vi "纳清浊度电极校准.vi"() -> ()   [LabVIEW 2016, in "斯坦道多参数.lvlib"]
uses:
  <vilib>/Utility/miscctls.llb/LVPointTypeDef.ctl
  <vilib>/Utility/miscctls.llb/LVPositionTypeDef.ctl
  <vilib>/Analysis/NI_AALBase.lvlib
panel:
  out "滤波设定":sgl
  out "第三点信号值":dbl
  out "第二点信号值":dbl
  out "第一点信号值":dbl
  in  "量程":u16(ring) items=["0-100", "0-500", "0-2000", "0-4000"]
  out "报警信息":string
  out "通讯状态":string
  out "第三点校准值":dbl
  out "标液3":sgl
  out "第二点校准值":dbl
  out "第一点校准值":dbl
  in  "校准停止":bool
  in  "校准启动":bool
  in  "校准模式":u16(ring)=1 items=["两点校准", "单点校准", "三点校准"]
  out "最小值":sgl format="%#.2f"
  out "最大值":sgl format="%#.2f"
  out "波形图表":dbl(graph) caption="历史曲线"
  out "mean":dbl caption="均值" format="%#.2f"
  out "standard deviation":dbl caption="标准差" format="%#.2f"
  out "变异系数":dbl format="%#.6f"
  out "测量值":sgl format="%#.2f"
  out "提示":string
  out "标液2":sgl
  out "标液1":sgl
  out "原始光强数值":u16 caption="信号值"
  out "温度":dbl format="%#.2f"
  # "浊度电极设定"
  # "℃"
  # "NTU"
  # "NTU"
  # "请选择校准模式:"
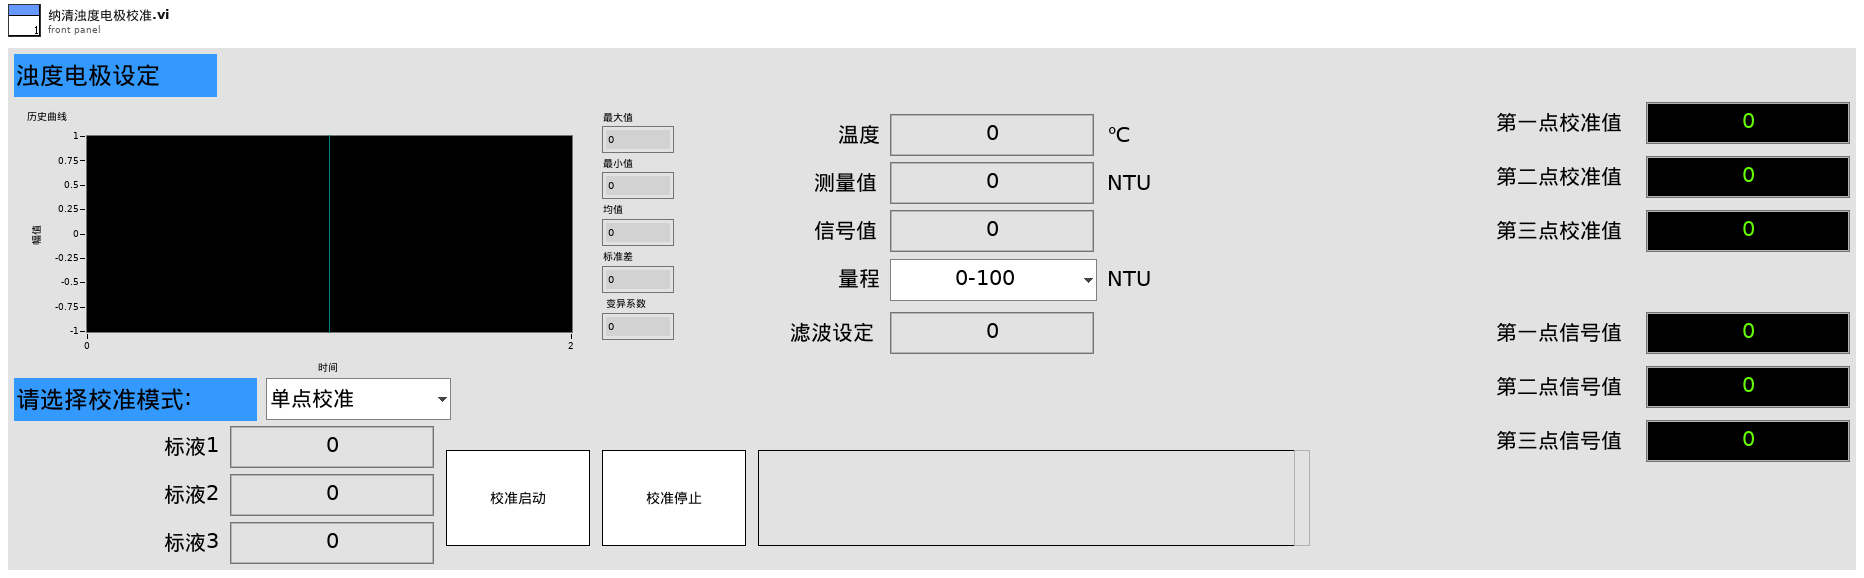
[diagram p1: front panel]
types:
  T1 = enum16{"pH", "DO", "Cond", "Turb", "ORP", "叶绿素a", "藻密度"}
  T2 = typedef "LVPointTypeDef.ctl" = cluster{"Horizontal":i16, "Vertical":i16}
  T3 = cluster{"报警码":u16, "浊度数值 NTU":sgl, "温度数据":sgl, "原始光强数值":u16, "量程":u16, "平均次数":u16, "清扫模式":u16, "清扫次数":u16, "清扫间隔分钟":u16, "0X000B_NC":string, "产品名称":string, "序列号":string, "硬件版本":string, "软件版本":string, "通讯地址":u16, "波特率":u16, "设备类型":u16, "0X0026_NC":string, "校准量程":u16, "第一点原始光强":u16, "第一点校准数据":sgl, "第二点原始光强":u16, "第二点校准数据":sgl, "第三点原始光强":u16, "第三点校准数据":sgl, "探头校准命令":u16, "温度校准参数":sgl, "温度校准命令":u16}
  T4 = cluster{"pH":u32, "DO":u32, "Cond":u32, "Turb":u32, "叶绿素a":u32, "藻密度":u32, "ORP":u32}
  T5 = typedef "LVPositionTypeDef.ctl" = cluster{"Left":i32, "Top":i32}
  T6 = enum8{"Enabled", "Disabled", "Disabled and Grayed Out"}
  T7 = cluster{"报警码":u16, "叶绿素a":sgl, "温度数据":sgl, "原始光强数值":u16, "量程":u16, "平均次数":u16, "清扫模式":u16, "清扫次数":u16, "清扫间隔分钟":u16, "0X000B_NC":string, "产品名称":string, "序列号":string, "硬件版本":string, "软件版本":string, "通讯地址":u16, "波特率":u16, "设备类型":u16, "0X0026_NC":string, "校准量程":u16, "第一点原始光强":u16, "第一点校准数据":sgl, "第二点原始光强":u16, "第二点校准数据":sgl, "第三点原始光强":u16, "第三点校准数据":sgl, "探头校准命令":u16, "温度校准参数":sgl, "温度校准命令":u16}
  T8 = cluster{"ph":bool, "DO":bool, "Cond":bool, "Turb":bool, "叶绿素a":bool, "藻密度":bool, "ORP":bool}
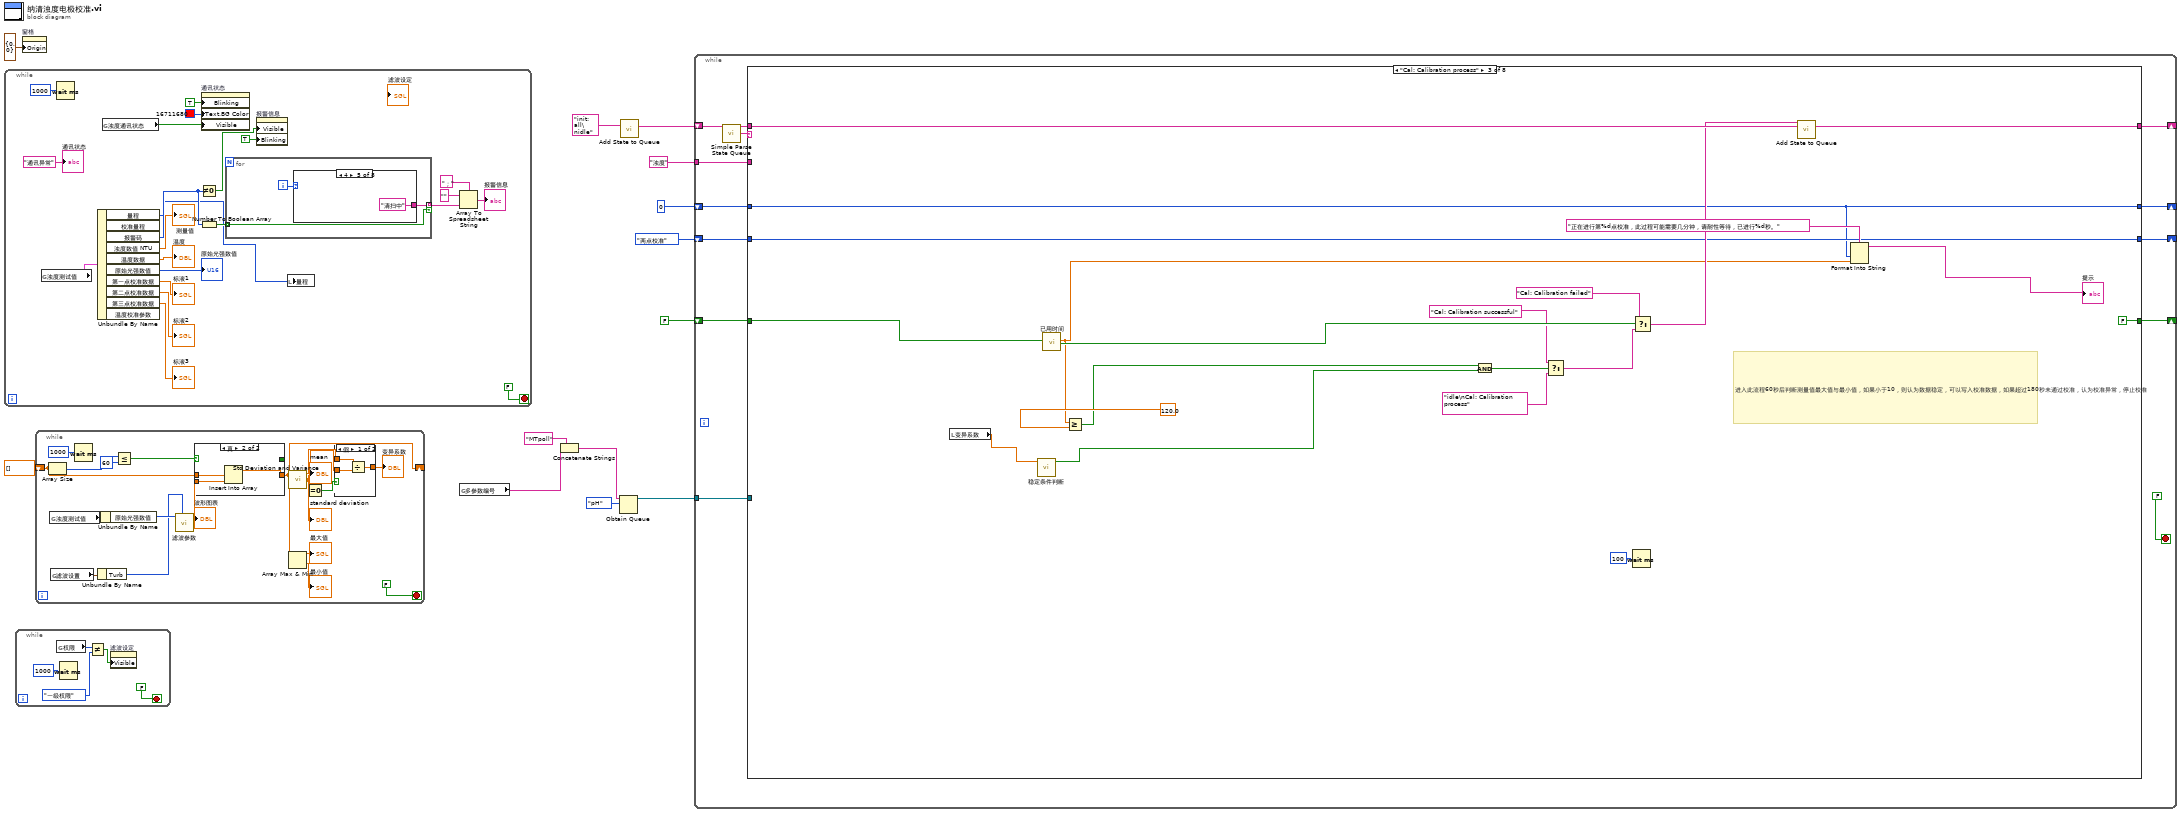
[diagram p0: block diagram]
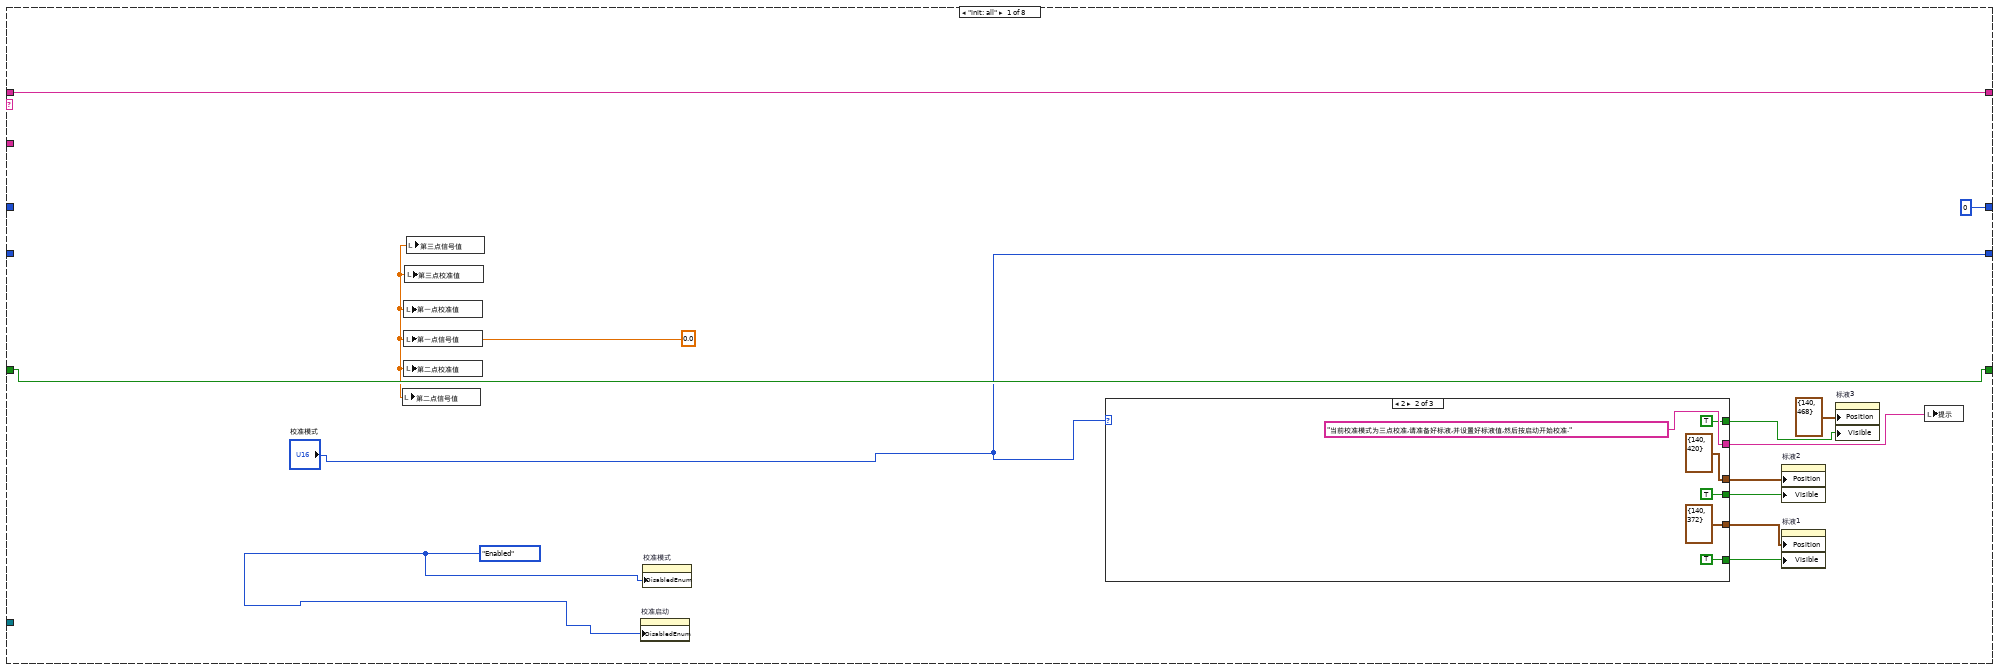
[diagram p2: hidden frame]
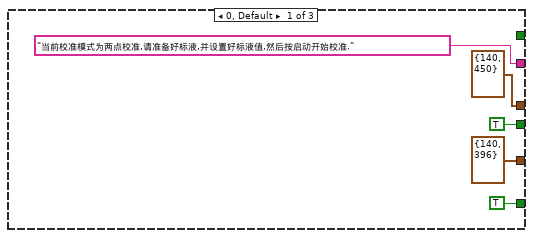
[diagram p3: hidden frame]
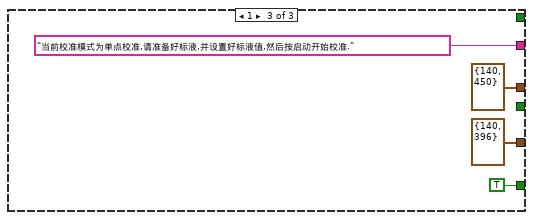
[diagram p4: hidden frame]
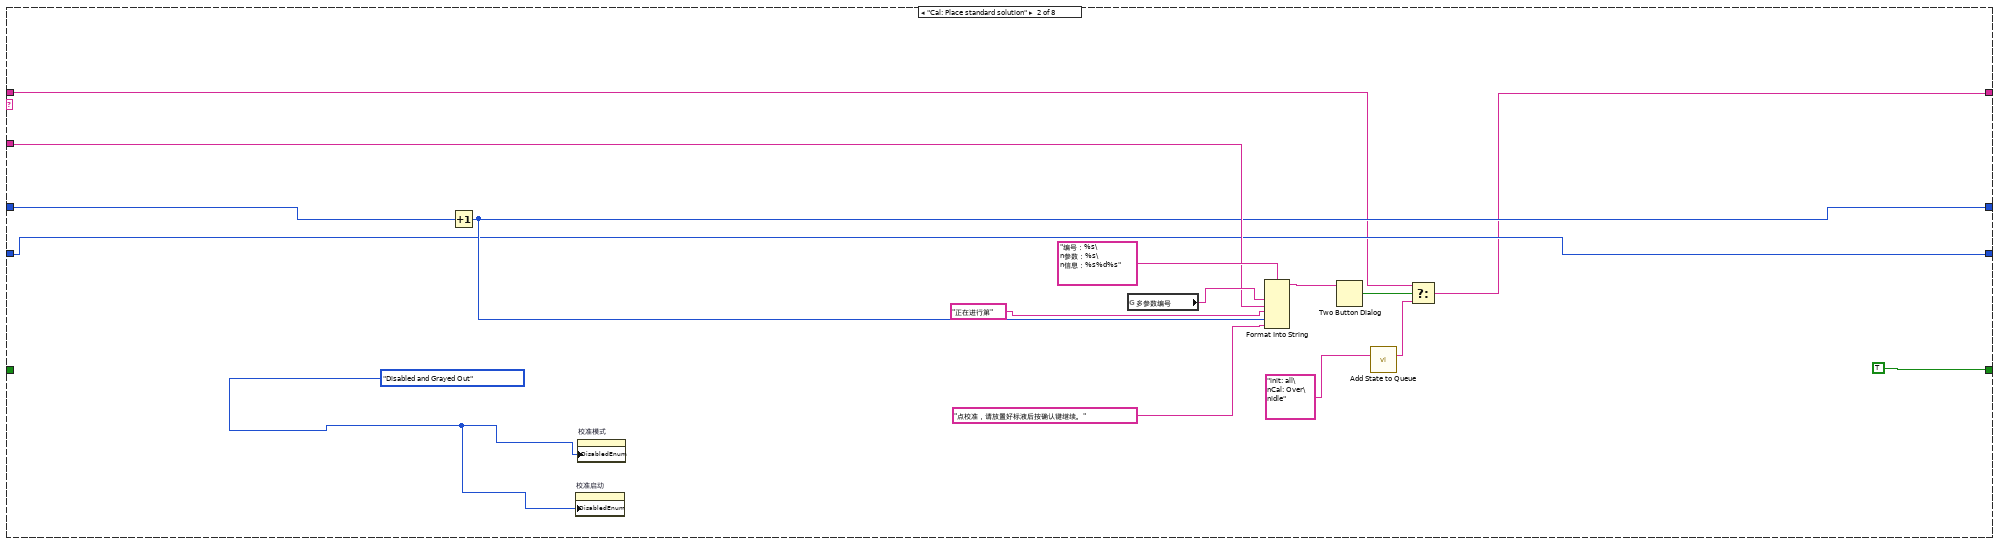
[diagram p5: hidden frame]
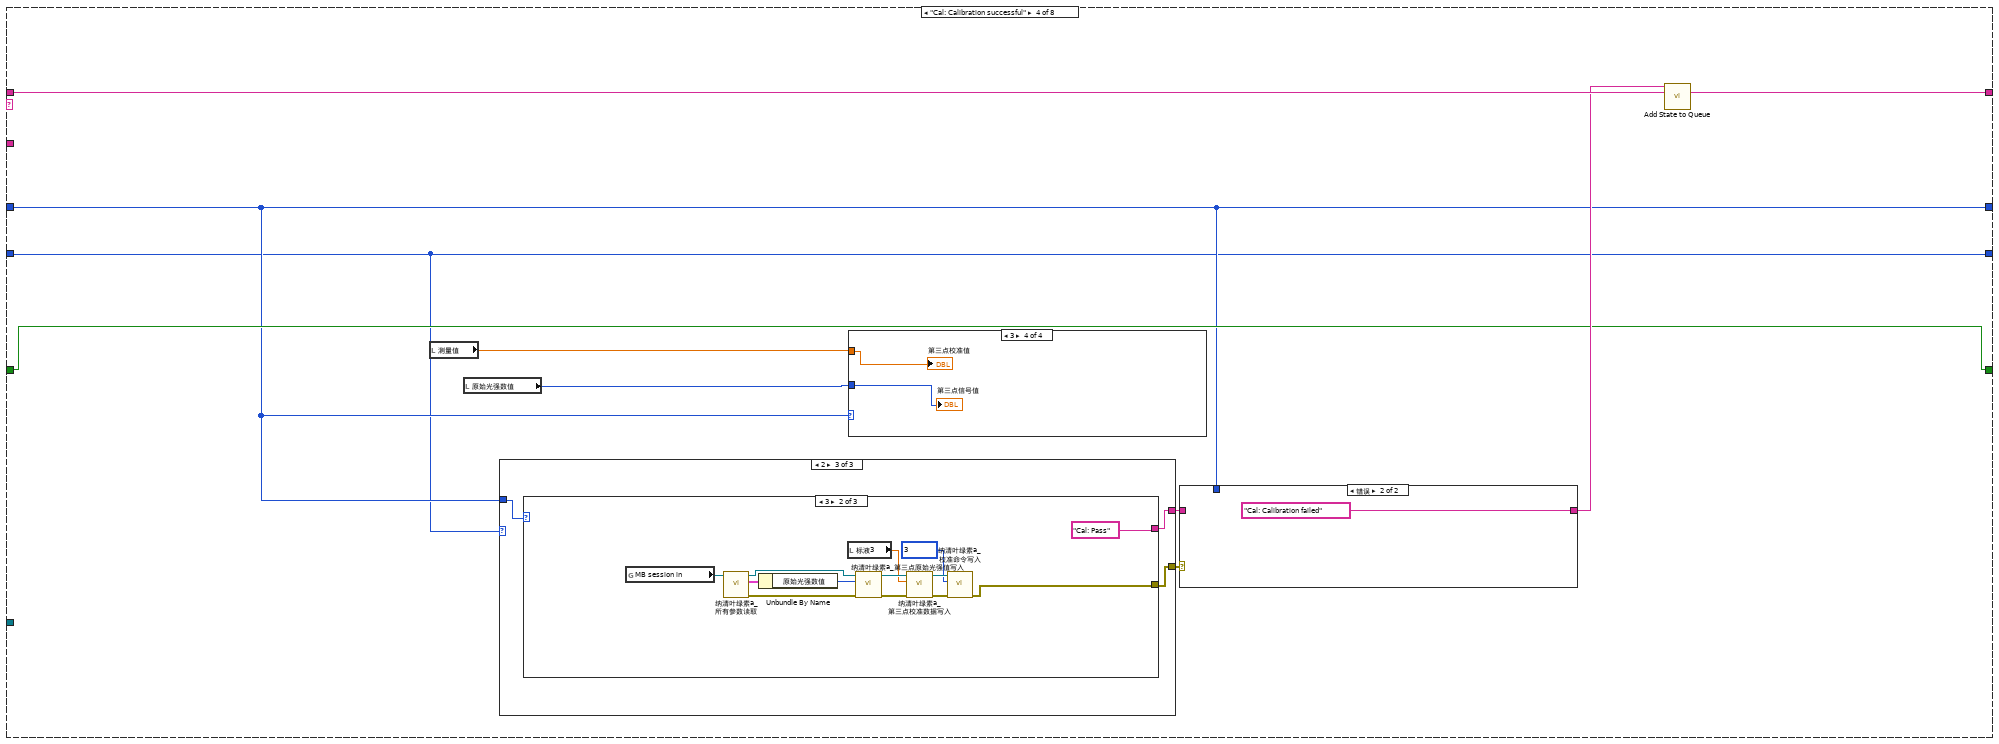
[diagram p6: hidden frame]
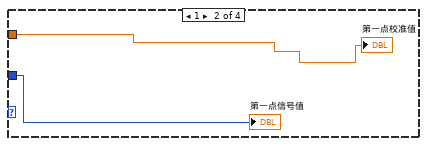
[diagram p8: hidden frame]
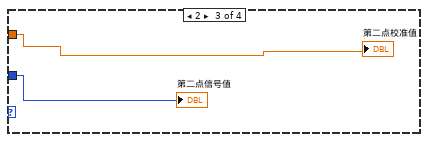
[diagram p9: hidden frame]
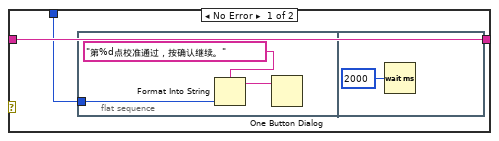
[diagram p10: hidden frame]
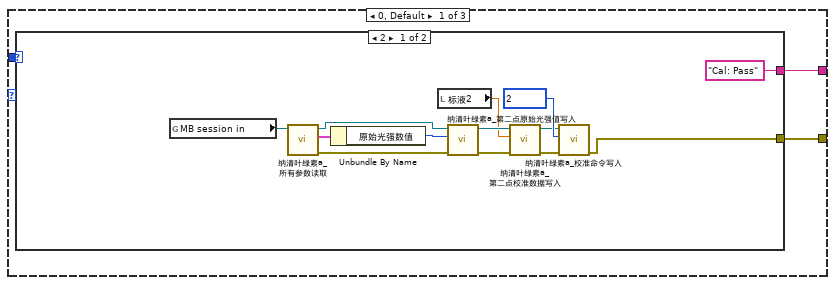
[diagram p11: hidden frame]
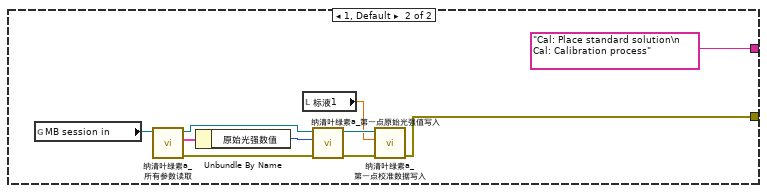
[diagram p12: hidden frame]
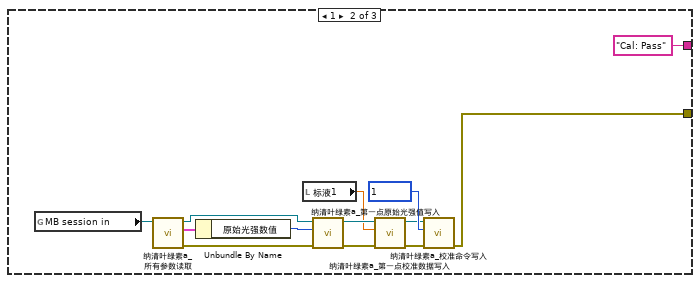
[diagram p13: hidden frame]
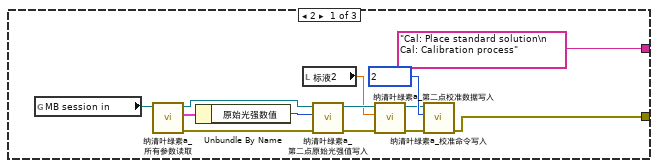
[diagram p14: hidden frame]
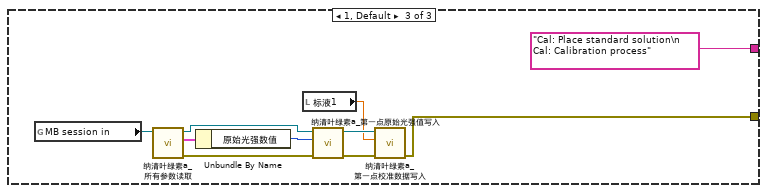
[diagram p15: hidden frame]
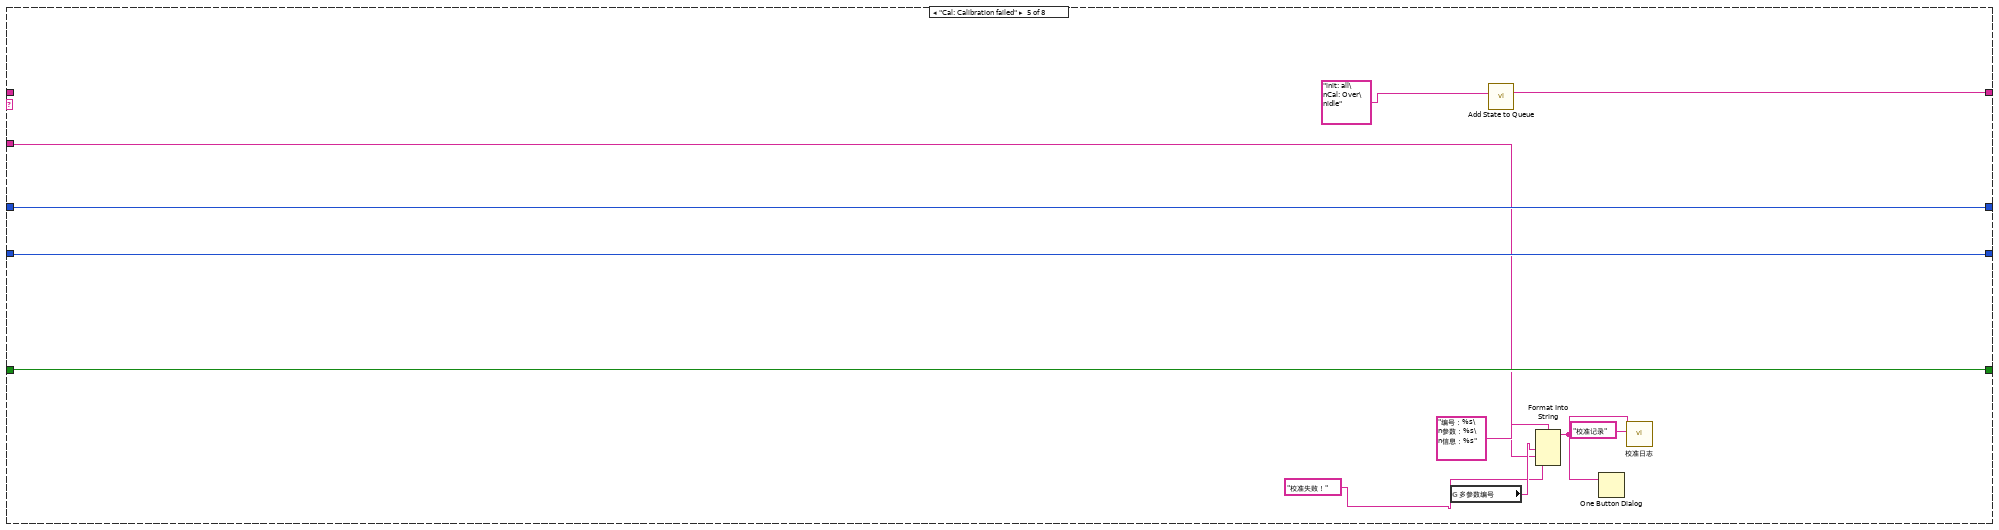
[diagram p16: hidden frame]
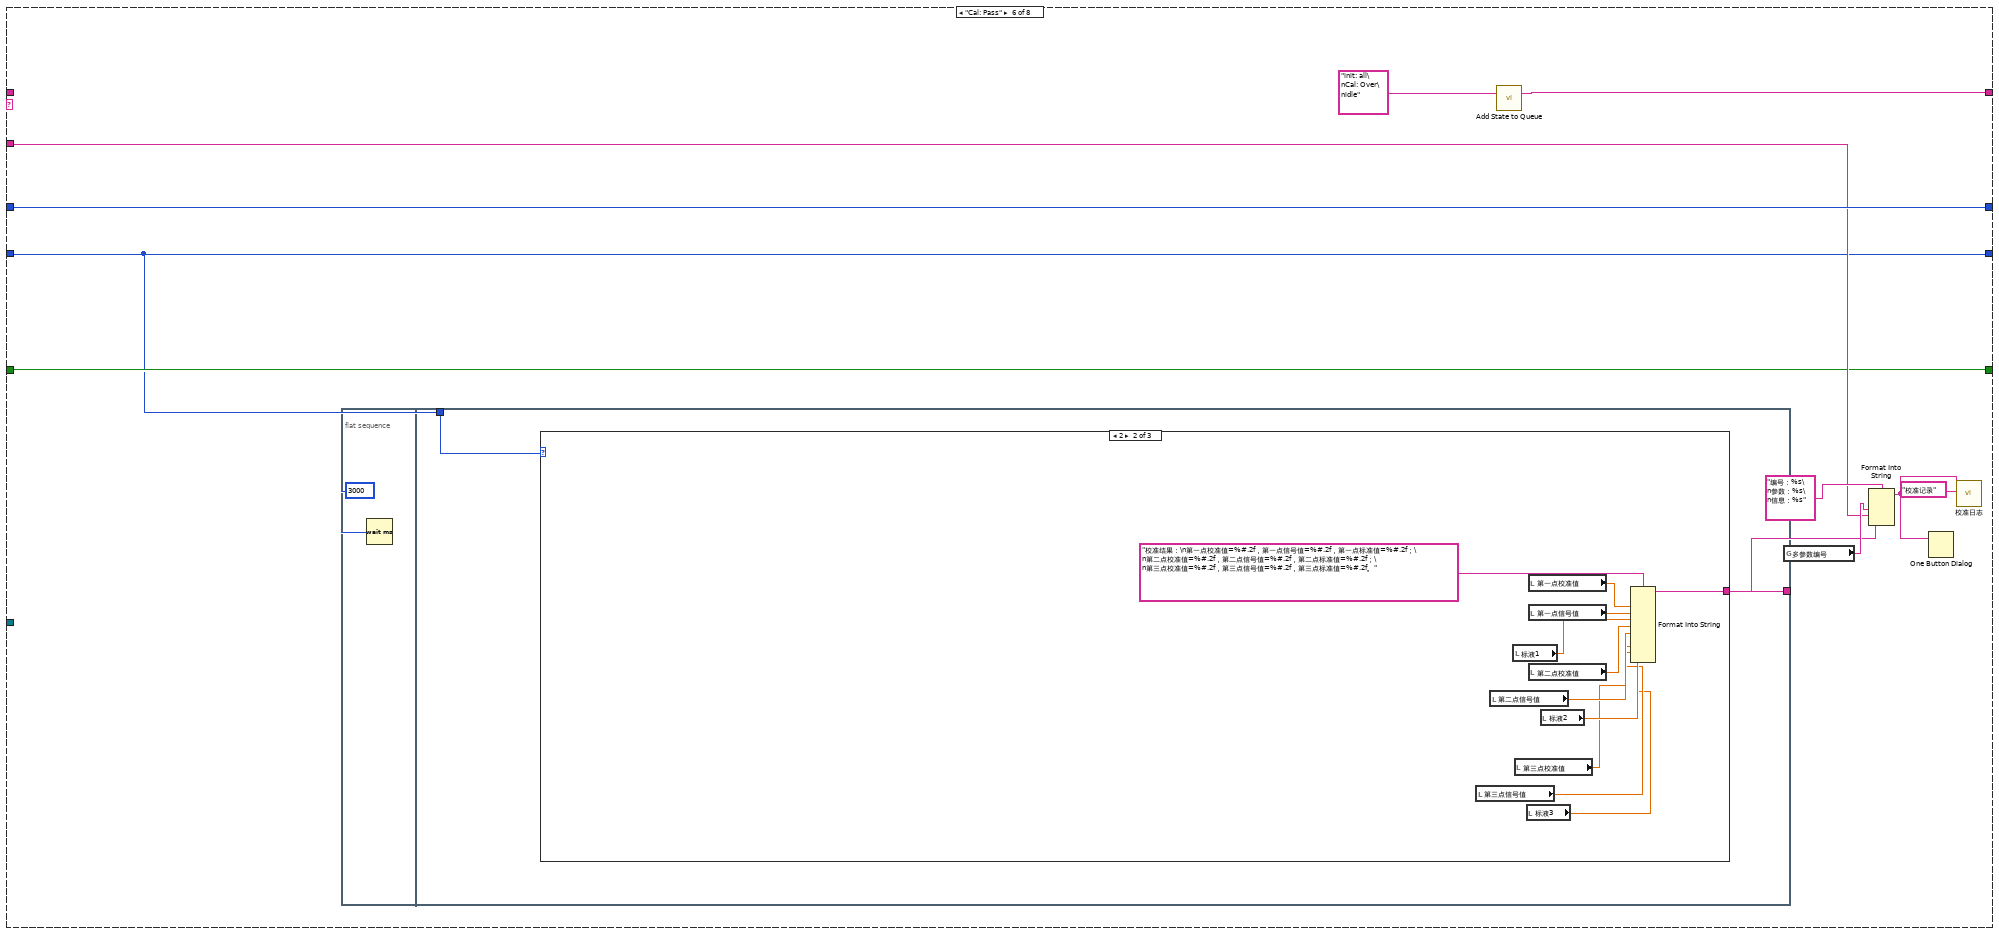
[diagram p17: hidden frame]
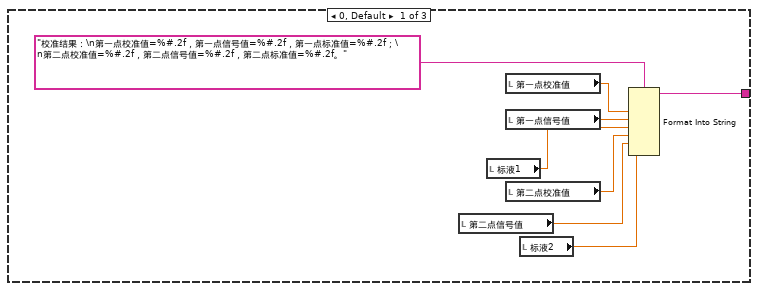
[diagram p18: hidden frame]
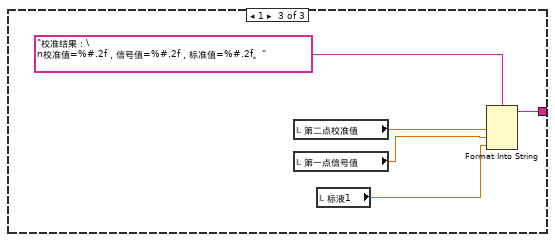
[diagram p19: hidden frame]
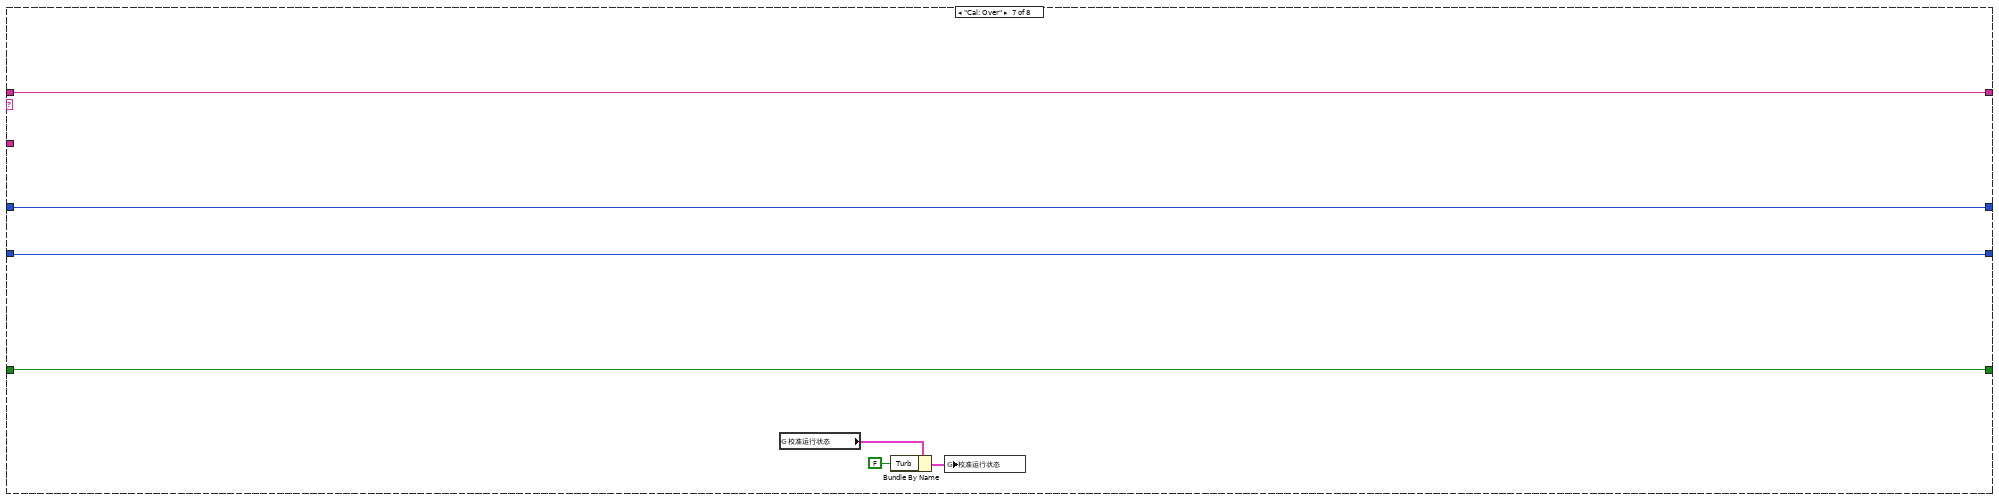
[diagram p20: hidden frame]
diagram:
  n1 = while {
    stop <- FALSE stop-if-true
    n2 = global read "纳清过程全局变量.vi" "浊度测试值"() -> (w33:T3)
    n3 = Wait (ms)(milliseconds to wait=u32 1000 ("等待时间（毫秒）")) -> ()  [unwired: 1 out]
    n4 = Unbundle By Name(w33) -> ("量程"=w14:u16, "报警码"=w15:u16, "浊度数值 NTU"=→"测量值":sgl, "温度数据"=→"温度":sgl, "原始光强数值"=→"原始光强数值":u16, "第一点校准数据"=→"标液1":sgl, "第二点校准数据"=→"标液2":sgl, "第三点校准数据"=→"标液3":sgl)  [unwired: 2 out]
    n5 = global read "多参数全局变量.vi" "浊度通讯状态"() -> (w23:bool)
    n6 = Not Equal To 0?(x=w15) -> (x != 0?=w17:bool)
    n7 = Number To Boolean Array(number=w15) -> (Boolean array=w22:bool[])
    n8 = property on="通讯状态" class="Str"("Blinking"=TRUE ("闪烁"), "Text.BG Color"=u32 16711680, "Visible"=w23) -> ()  [unwired: 2 in, 2 out]
    n9 = for {
      tunnel: w22 -> [w36] mode=indexing
      tunnel: [w37] -> w21 mode=indexing if=w36
      i -> [w38]
      n10 = case shown="4" w38 {
        tunnel: [_ "浊度超量程" "温度超量程" "光强信号超范围" "清扫中" "温度传感器故障" "电极故障" "内部电压基准故障"] -> w37
        frame Default {
        }
        frame 0 {
        }
        frame 2 {
        }
        frame 3 {
        }
        frame 4 {
        }
        frame 8 {
        }
        frame 9 {
        }
        frame 10 {
        }
      }
    }
    n11 = property on="报警信息" class="Str"("Visible"=w17, "Blinking"=TRUE ("闪烁")) -> ()  [unwired: 2 in, 2 out]
    n12 = local write "量程"(w14) -> ()
    n13 = Array To Spreadsheet String(delimiter (Tab)="；" ("分隔符(Tab)"), array=w21, 3:"" ("格式字符串")) -> (spreadsheet string=→"报警信息":string)
    "通讯状态" <- "通讯异常" ("当前串口")
  }
  n14 = while {
    stop <- FALSE stop-if-true
    n15 = global read "多参数全局变量.vi" "权限"() -> (w49:enum16{"一级权限", "二级权限", "三级权限"})
    n16 = Wait (ms)(milliseconds to wait=u32 1000 ("等待时间（毫秒）")) -> ()  [unwired: 1 out]
    n17 = Not Equal?(x=w49, y=enum16{"一级权限", "二级权限", "三级权限"}."一级权限") -> (x != y?=w46:bool)
    n18 = property on="滤波设定" class="DigNum (严格)"("Visible"=w46) -> ()  [unwired: 2 in, 2 out]
  }
  n19 = property on="窗格" class="Pane"("Origin"=T2 {"Horizontal"=0, "Vertical"=0} ("原点")) -> ()  [unwired: 2 in, 2 out]
  n20 = while {
    shift-right: [w58] -> _
    shift-left: sgl[] [] -> [w64]
    stop <- FALSE stop-if-true
    n21 = Array Size(array=w64) -> (size(s)=w66:i32)
    n22 = global read "纳清过程全局变量.vi" "浊度测试值"() -> (w55:T3)
    n23 = global read "断电保存变量.vi" "滤波设置"() -> (w52:T4)
    n24 = Wait (ms)(milliseconds to wait=u32 1000 ("等待时间（毫秒）")) -> ()  [unwired: 1 out]
    n25 = Unbundle By Name(w52) -> ("Turb"=w51:u32)
    n26 = Unbundle By Name(w55) -> ("原始光强数值"=w54:u16)
    n27 = Less Or Equal?(x=w66, y=60) -> (x <= y?=w65:bool)
    n28 = call "滤波参数.vi"("滤波次数"=w51, "x"=w54) -> ("mode"=w53:dbl)  [unwired: 9 in]
    "波形图表" <- w53
    n29 = case shown="真" w65 {
      tunnel: w64 -> [w77 w80]
      tunnel: w53 -> [w75 w79]
      tunnel: [w73 w78] -> w58
      tunnel: [TRUE _] -> _
      frame False {
        n30 = Replace Array Subset(array=w77, new element=w75) -> (w76:sgl[])  [unwired: 1 in]
        n31 = Rotate 1D Array(1:w76, 2:-1 ("n")) -> (0:w73:sgl[])
      }
      frame True {
        n32 = Insert Into Array(array=w80, new element=w79) -> (w78:sgl[])  [unwired: 1 in]
      }
    }
    n33 = call <vilib>:"Std Deviation and Variance.vi"("X"=w58) -> ("mean"=w62:dbl, "standard deviation"=w61:dbl)  [unwired: 1 in, 1 out]
    "mean" <- w62
    "standard deviation" <- w61
    n34 = Array Max & Min(array=w58) -> (max value=→"最大值":sgl, min value=→"最小值":sgl)  [unwired: 2 out]
    n35 = Equal To 0?(x=w62) -> (x = 0?=w63:bool)
    n36 = case shown="假" w63 {
      tunnel: w61 -> [w71 _]
      tunnel: [w70 _] -> w60
      tunnel: w62 -> [w69 _]
      frame False {
        n37 = Divide(x=w71, y=w69) -> (x/y=w70:dbl)
      }
      frame True {
      }
    }
    "变异系数" <- w60
  }
  n38 = global read "多参数全局变量.vi" "多参数编号"() -> (w2:string)
  n39 = Concatenate Strings("MTpoll" ("名称（未命名）"), w2) -> (w4:string)
  n40 = Obtain Queue(name (unnamed)=w4, element data type=T1."pH" ("枚举")) -> (queue out=w1:refnum<queue>)  [unwired: 3 in, 2 out]
  n41 = call "Add State to Queue.vi"("State(s) In (\"\")"="init: all\nidle" ("State(s) In (\"\")")) -> ("States Out"=w10:string)  [unwired: 14 in]
  n42 = while {
    shift-right: [w89] -> _
    shift-left: w10 -> [w93]
    shift-right: [w86] -> _
    shift-left: 0 -> [w88]
    tunnel: "浊度" ("State(s) In (\"\")") -> [w87]
    shift-right: [w84] -> _
    shift-left: enum16{"两点校准", "单点校准", "三点校准"}."两点校准" ("校准模式") -> [w85]
    shift-right: [w82] -> _
    shift-left: FALSE -> [w83]
    tunnel: w1 -> [w81]
    stop <- FALSE stop-if-true
    n43 = call "Simple Parse State Queue.vi"("State Queue"=w93) -> ("Remain States"=w90:string, "Next State"=w91:string)  [unwired: 13 in]
    n44 = case shown="\"Cal: Calibration process\"" w91 {
      tunnel: w90 -> [w106 w125 w157 w166 _ _ w315 w323]
      tunnel: [w106 w124 w156 w165 w267 w272 w315 w322] -> w89
      tunnel: w88 -> [_ w133 w142 w160 w270 w281 w314 w320]
      tunnel: w87 -> [_ w134 _ _ w261 w277 _ _]
      tunnel: [0 w131 w142 w160 w270 w281 w314 w321] -> w86
      tunnel: w85 -> [_ w130 w143 w159 w269 w273 w313 w319]
      tunnel: ["校准模式" w130 w143 w159 w269 w273 w313 w319] -> w84
      tunnel: w83 -> [w104 _ w145 w161 w268 w276 w312 w317]
      tunnel: [w104 TRUE FALSE w161 w268 w276 w312 w317] -> w82
      tunnel: w81 -> [_ _ _ _ _ _ _ w316]
      frame "init: all" {
        w102 = T6."Enabled" ("禁用")
        w103 = 0.0 ("第一点校准值")
        n45 = local write "第二点信号值"(w103) -> ()
        n46 = local write "第一点校准值"(w103) -> ()
        n47 = local write "第一点信号值"(w103) -> ()
        n48 = local write "第二点校准值"(w103) -> ()
        n49 = local write "第三点校准值"(w103) -> ()
        n50 = local write "第三点信号值"(w103) -> ()
        n51 = property on="校准启动" class="Bool"("DisabledEnum"=w102) -> ()  [unwired: 2 in, 2 out]
        n52 = property on="校准模式" class="Ring (严格)"("DisabledEnum"=w102) -> ()  [unwired: 2 in, 2 out]
        n53 = case shown="2" "校准模式" {
          tunnel: ["当前校准模式为两点校准,请准备好标液,并设置好标液值,然后按启动开始校准." ("提示") "当前校准模式为三点校准,请准备好标液,并设置好标液值,然后按启动开始校准." ("提示") "当前校准模式为单点校准,请准备好标液,并设置好标液值,然后按启动开始校准." ("提示")] -> w94
          tunnel: [TRUE ("可见") TRUE ("可见") _] -> w99
          tunnel: [T5 {"Left"=140, "Top"=396} ("位置") T5 {"Left"=140, "Top"=372} ("位置") T5 {"Left"=140, "Top"=396} ("位置")] -> w96
          tunnel: [T5 {"Left"=140, "Top"=450} ("位置 2") T5 {"Left"=140, "Top"=420} ("位置 2") T5 {"Left"=140, "Top"=450} ("位置 2")] -> w97
          tunnel: [_ TRUE ("可见") _] -> w100
          tunnel: [TRUE ("可见") TRUE ("可见") TRUE ("可见")] -> w101
          frame 0, Default {
          }
          frame 2 {
          }
          frame 1 {
          }
        }
        n54 = property on="标液2" class="DigNum (严格)"("Position"=w97, "Visible"=w99) -> ()  [unwired: 2 in, 2 out]
        n55 = property on="标液1" class="DigNum (严格)"("Position"=w96, "Visible"=w101) -> ()  [unwired: 2 in, 2 out]
        n56 = property on="标液3" class="DigNum (严格)"("Position"=T5 {"Left"=140, "Top"=468} ("位置 3"), "Visible"=w100) -> ()  [unwired: 2 in, 2 out]
        n57 = local write "提示"(w94) -> ()
      }
      frame "Cal: Place standard solution" {
        w123 = T6."Disabled and Grayed Out" ("禁用")
        n58 = Increment(x=w133) -> (x+1=w131:i32)
        n59 = property on="校准启动" class="Bool"("DisabledEnum"=w123) -> ()  [unwired: 2 in, 2 out]
        n60 = property on="校准模式" class="Ring (严格)"("DisabledEnum"=w123) -> ()  [unwired: 2 in, 2 out]
        n61 = global read "多参数全局变量.vi" "多参数编号"() -> (w136:string)
        n62 = Format Into String(format string="编号：%s\n参数：%s\n信息：%s%d%s" ("格式字符串"), w136, w134, "正在进行第" ("消息"), w131, "点校准，请放置好标液后按确认键继续。" ("消息")) -> (resulting string=w128:string)  [unwired: 2 in, 1 out]
        n63 = Two Button Dialog(message=w128) -> (T button?=w127:bool)  [unwired: 2 in]
        n64 = call "Add State to Queue.vi"("State(s) In (\"\")"="init: all\nCal: Over\nidle" ("State(s) In (\"\")")) -> ("States Out"=w126:string)  [unwired: 14 in]
        n65 = Select(t=w125, s=w127, f=w126) -> (s? t:f=w124:string)
      }
      frame "Cal: Calibration process" {
        # "进入此流程60秒后判断测量值最大值与最小值，如果小于10，则认为数据稳定，可以写入校准数据，如果超过180秒未通过校准，认为校准异常，停止校准"
        n66 = local read "变异系数"() -> (w139:dbl)
        n67 = call "稳定条件判断.vi"("变异系数"=w139) -> ("布尔"=w138:bool)  [unwired: 10 in]
        n68 = call "已用时间"("Reset"=w145) -> ("Elapsed Time (s)"=w141:dbl, "Time has Elapsed"=w158:bool)  [unwired: 11 in, 6 out]
        n69 = Greater Or Equal?(x=w141, y=120.0) -> (x >= y?=w153:bool)
        n70 = And(x=w153, y=w138) -> (x .and. y?=w150:bool)
        n71 = Select(t="Cal: Calibration successful" ("State(s) In (\"\")"), s=w150, f="idle\nCal: Calibration process" ("State(s) In (\"\")")) -> (s? t:f=w149:string)
        n72 = Wait (ms)(milliseconds to wait=u32 100 ("等待时间（毫秒）")) -> ()  [unwired: 1 out]
        n73 = Select(t="Cal: Calibration failed" ("State(s) In (\"\")"), s=w158, f=w149) -> (s? t:f=w148:string)
        n74 = call "Add State to Queue.vi"("State(s) In Front (\"\")"=w148, "State(s) In (\"\")"=w157) -> ("States Out"=w156:string)  [unwired: 13 in]
        n75 = Format Into String(format string="正在进行第%d点校准，此过程可能需要几分钟，请耐性等待，已进行%d秒。" ("格式字符串"), w142, w141) -> (resulting string=→"提示":string)  [unwired: 2 in, 1 out]
      }
      frame "Cal: Calibration successful" {
        n76 = local read "测量值"() -> (w162:sgl)
        n77 = local read "原始光强数值"() -> (w163:u16)
        n78 = case shown="2" w159 {
          tunnel: [w184 w208 w221] -> w168
          tunnel: [w183 "Cal: Pass" ("State(s) In (\"\")") w222] -> w167
          tunnel: w160 -> [w182 _ w223]
          frame 0, Default {
            n79 = case shown="2" w182 {
              tunnel: [w185 w198] -> w184
              tunnel: ["Cal: Pass" ("State(s) In (\"\")") "Cal: Place standard solution\n Cal: Calibration process" ("State(s) In (\"\")")] -> w183
              frame 2 {
                n80 = global read "多参数全局变量.vi" "MB session in"() -> (w193:refnum<class "MB_Master.lvclass">)
                n81 = call "纳清叶绿素a_所有参数读取.vi"("MB session in"=w193) -> ("error out"=w195:errorcluster, "输出值"=w192:T7, "MB session out"=w194:refnum<class "MB_Master.lvclass">)  [unwired: 8 in]
                n82 = Unbundle By Name(w192) -> ("原始光强数值"=w191:u16)
                n83 = local read "标液2"() -> (w186:sgl)
                n84 = call "纳清叶绿素a_第二点原始光强值写入.vi"("error in (no error)"=w195, "数值"=w191, "MB session in"=w194) -> ("error out"=w190:errorcluster, "MB session out"=w189:refnum<class "MB_Master.lvclass">)  [unwired: 7 in]
                n85 = call "纳清叶绿素a_第二点校准数据写入.vi"("error in (no error)"=w190, "数值"=w186, "MB session in"=w189) -> ("error out"=w188:errorcluster, "MB session out"=w187:refnum<class "MB_Master.lvclass">)  [unwired: 7 in]
                n86 = call "纳清叶绿素a_校准命令写入.vi"("error in (no error)"=w188, "数值"=u16 2 ("starting address"), "MB session in"=w187) -> ("error out"=w185:errorcluster)  [unwired: 7 in, 1 out]
              }
              frame 1, Default {
                n87 = global read "多参数全局变量.vi" "MB session in"() -> (w204:refnum<class "MB_Master.lvclass">)
                n88 = call "纳清叶绿素a_所有参数读取.vi"("MB session in"=w204) -> ("error out"=w206:errorcluster, "输出值"=w203:T7, "MB session out"=w205:refnum<class "MB_Master.lvclass">)  [unwired: 8 in]
                n89 = Unbundle By Name(w203) -> ("原始光强数值"=w202:u16)
                n90 = local read "标液1"() -> (w199:sgl)
                n91 = call "纳清叶绿素a_第一点原始光强值写入.vi"("error in (no error)"=w206, "数值"=w202, "MB session in"=w205) -> ("error out"=w201:errorcluster, "MB session out"=w200:refnum<class "MB_Master.lvclass">)  [unwired: 7 in]
                n92 = call "纳清叶绿素a_第一点校准数据写入.vi"("error in (no error)"=w201, "数值"=w199, "MB session in"=w200) -> ("error out"=w198:errorcluster)  [unwired: 7 in, 1 out]
              }
            }
          }
          frame 1 {
            n93 = global read "多参数全局变量.vi" "MB session in"() -> (w216:refnum<class "MB_Master.lvclass">)
            n94 = call "纳清叶绿素a_所有参数读取.vi"("MB session in"=w216) -> ("error out"=w218:errorcluster, "输出值"=w215:T7, "MB session out"=w217:refnum<class "MB_Master.lvclass">)  [unwired: 8 in]
            n95 = Unbundle By Name(w215) -> ("原始光强数值"=w214:u16)
            n96 = local read "标液1"() -> (w209:sgl)
            n97 = call "纳清叶绿素a_第一点原始光强值写入.vi"("error in (no error)"=w218, "数值"=w214, "MB session in"=w217) -> ("error out"=w213:errorcluster, "MB session out"=w212:refnum<class "MB_Master.lvclass">)  [unwired: 7 in]
            n98 = call "纳清叶绿素a_第一点校准数据写入.vi"("error in (no error)"=w213, "数值"=w209, "MB session in"=w212) -> ("error out"=w211:errorcluster, "MB session out"=w210:refnum<class "MB_Master.lvclass">)  [unwired: 7 in]
            n99 = call "纳清叶绿素a_校准命令写入.vi"("error in (no error)"=w211, "数值"=u16 1 ("starting address"), "MB session in"=w210) -> ("error out"=w208:errorcluster)  [unwired: 7 in, 1 out]
          }
          frame 2 {
            n100 = case shown="3" w223 {
              tunnel: [w225 w237 w250] -> w221
              tunnel: ["Cal: Place standard solution\n Cal: Calibration process" ("State(s) In (\"\")") "Cal: Pass" ("State(s) In (\"\")") "Cal: Place standard solution\n Cal: Calibration process" ("State(s) In (\"\")")] -> w222
              frame 2 {
                n101 = global read "多参数全局变量.vi" "MB session in"() -> (w233:refnum<class "MB_Master.lvclass">)
                n102 = call "纳清叶绿素a_所有参数读取.vi"("MB session in"=w233) -> ("error out"=w235:errorcluster, "输出值"=w232:T7, "MB session out"=w234:refnum<class "MB_Master.lvclass">)  [unwired: 8 in]
                n103 = Unbundle By Name(w232) -> ("原始光强数值"=w231:u16)
                n104 = local read "标液2"() -> (w226:sgl)
                n105 = call "纳清叶绿素a_第二点原始光强值写入.vi"("error in (no error)"=w235, "数值"=w231, "MB session in"=w234) -> ("error out"=w230:errorcluster, "MB session out"=w229:refnum<class "MB_Master.lvclass">)  [unwired: 7 in]
                n106 = call "纳清叶绿素a_第二点校准数据写入.vi"("error in (no error)"=w230, "数值"=w226, "MB session in"=w229) -> ("error out"=w228:errorcluster, "MB session out"=w227:refnum<class "MB_Master.lvclass">)  [unwired: 7 in]
                n107 = call "纳清叶绿素a_校准命令写入.vi"("error in (no error)"=w228, "数值"=u16 2 ("starting address"), "MB session in"=w227) -> ("error out"=w225:errorcluster)  [unwired: 7 in, 1 out]
              }
              frame 3 {
                n108 = global read "多参数全局变量.vi" "MB session in"() -> (w246:refnum<class "MB_Master.lvclass">)
                n109 = call "纳清叶绿素a_所有参数读取.vi"("MB session in"=w246) -> ("error out"=w248:errorcluster, "输出值"=w245:T7, "MB session out"=w247:refnum<class "MB_Master.lvclass">)  [unwired: 8 in]
                n110 = Unbundle By Name(w245) -> ("原始光强数值"=w244:u16)
                n111 = local read "标液3"() -> (w238:sgl)
                n112 = call "纳清叶绿素a_第三点原始光强值写入.vi"("error in (no error)"=w248, "数值"=w244, "MB session in"=w247) -> ("error out"=w243:errorcluster, "MB session out"=w242:refnum<class "MB_Master.lvclass">)  [unwired: 7 in]
                n113 = call "纳清叶绿素a_第三点校准数据写入.vi"("error in (no error)"=w243, "数值"=w238, "MB session in"=w242) -> ("error out"=w241:errorcluster, "MB session out"=w240:refnum<class "MB_Master.lvclass">)  [unwired: 7 in]
                n114 = call "纳清叶绿素a_校准命令写入.vi"("error in (no error)"=w241, "数值"=u16 3 ("starting address"), "MB session in"=w240) -> ("error out"=w237:errorcluster)  [unwired: 7 in, 1 out]
              }
              frame 1, Default {
                n115 = global read "多参数全局变量.vi" "MB session in"() -> (w256:refnum<class "MB_Master.lvclass">)
                n116 = call "纳清叶绿素a_所有参数读取.vi"("MB session in"=w256) -> ("error out"=w258:errorcluster, "输出值"=w255:T7, "MB session out"=w257:refnum<class "MB_Master.lvclass">)  [unwired: 8 in]
                n117 = Unbundle By Name(w255) -> ("原始光强数值"=w254:u16)
                n118 = local read "标液1"() -> (w251:sgl)
                n119 = call "纳清叶绿素a_第一点原始光强值写入.vi"("error in (no error)"=w258, "数值"=w254, "MB session in"=w257) -> ("error out"=w253:errorcluster, "MB session out"=w252:refnum<class "MB_Master.lvclass">)  [unwired: 7 in]
                n120 = call "纳清叶绿素a_第一点校准数据写入.vi"("error in (no error)"=w253, "数值"=w251, "MB session in"=w252) -> ("error out"=w250:errorcluster)  [unwired: 7 in, 1 out]
              }
            }
          }
        }
        n121 = case shown="3" w160 {
          tunnel: w163 -> [_ w170 w172 w173]
          tunnel: w162 -> [_ w169 w171 w174]
          frame 0, Default {
          }
          frame 1 {
            "第一点信号值" <- w170
            "第一点校准值" <- w169
          }
          frame 2 {
            "第二点信号值" <- w172
            "第二点校准值" <- w171
          }
          frame 3 {
            "第三点校准值" <- w174
            "第三点信号值" <- w173
          }
        }
        n122 = case shown="错误" w168 {
          tunnel: w167 -> [w176 _]
          tunnel: [w176 "Cal: Calibration failed" ("State(s) In (\"\")")] -> w164
          tunnel: w160 -> [w175 _]
          frame No Error {
            n123 = flat-sequence {
              tunnel: w175 -> [w177]
              frame #0 {
                n124 = Format Into String(format string="第%d点校准通过，按确认继续。" ("格式字符串"), w177) -> (resulting string=w179:string)  [unwired: 2 in, 1 out]
                n125 = One Button Dialog(message=w179) -> ()  [unwired: 1 in, 1 out]
              }
              frame #1 {
                n126 = Wait (ms)(milliseconds to wait=u32 2000 ("等待时间（毫秒）")) -> ()  [unwired: 1 out]
              }
            }
          }
          frame Error {
          }
        }
        n127 = call "Add State to Queue.vi"("State(s) In Front (\"\")"=w164, "State(s) In (\"\")"=w166) -> ("States Out"=w165:string)  [unwired: 13 in]
      }
      frame "Cal: Calibration failed" {
        n128 = global read "多参数全局变量.vi" "多参数编号"() -> (w264:string)
        n129 = call "Add State to Queue.vi"("State(s) In (\"\")"="init: all\nCal: Over\nidle" ("State(s) In (\"\")")) -> ("States Out"=w267:string)  [unwired: 14 in]
        n130 = Format Into String(format string="编号：%s\n参数：%s\n信息：%s" ("格式字符串"), w264, w261, "校准失败！" ("消息")) -> (resulting string=w263:string)  [unwired: 2 in, 1 out]
        n131 = One Button Dialog(message=w263) -> ()  [unwired: 1 in, 1 out]
        n132 = call "校准日志.vi"("table"="校准记录", "日志信息"=w263) -> ()  [unwired: 9 in, 1 out]
      }
      frame "Cal: Pass" {
        n133 = flat-sequence {
          tunnel: [w284] -> w274
          tunnel: w273 -> [w283]
          frame #0 {
            n134 = Wait (ms)(milliseconds to wait=u32 3000 ("等待时间（毫秒）")) -> ()  [unwired: 1 out]
          }
          frame #1 {
            n135 = case shown="2" w283 {
              tunnel: [w292 w303 w308] -> w284
              frame 0, Default {
                n136 = local read "第二点信号值"() -> (w286:dbl)
                n137 = local read "标液1"() -> (w288:sgl)
                n138 = local read "第一点校准值"() -> (w290:dbl)
                n139 = local read "第一点信号值"() -> (w291:dbl)
                n140 = local read "第二点校准值"() -> (w287:dbl)
                n141 = local read "标液2"() -> (w285:sgl)
                n142 = Format Into String(format string="校准结果：\n第一点校准值=%#.2f，第一点信号值=%#.2f，第一点标准值=%#.2f；\n第二点校准值=%#.2f，第二点信号值=%#.2f，第二点标准值=%#.2f。" ("提示"), w290, w291, w288, w287, w286, w285) -> (resulting string=w292:string)  [unwired: 2 in, 1 out]
              }
              frame 2 {
                n143 = local read "第三点信号值"() -> (w294:dbl)
                n144 = local read "第二点信号值"() -> (w297:dbl)
                n145 = local read "标液1"() -> (w299:sgl)
                n146 = local read "第三点校准值"() -> (w295:dbl)
                n147 = local read "标液3"() -> (w293:sgl)
                n148 = local read "第一点校准值"() -> (w301:dbl)
                n149 = local read "第一点信号值"() -> (w302:dbl)
                n150 = local read "第二点校准值"() -> (w298:dbl)
                n151 = local read "标液2"() -> (w296:sgl)
                n152 = Format Into String(format string="校准结果：\n第一点校准值=%#.2f，第一点信号值=%#.2f，第一点标准值=%#.2f；\n第二点校准值=%#.2f，第二点信号值=%#.2f，第二点标准值=%#.2f；\n第三点校准值=%#.2f，第三点信号值=%#.2f，第三点标准值=%#.2f。" ("提示"), w301, w302, w299, w298, w297, w296, w295, w294, w293) -> (resulting string=w303:string)  [unwired: 2 in, 1 out]
              }
              frame 1 {
                n153 = local read "第二点校准值"() -> (w307:dbl)
                n154 = local read "第一点信号值"() -> (w305:dbl)
                n155 = local read "标液1"() -> (w304:sgl)
                n156 = Format Into String(format string="校准结果：\n校准值=%#.2f，信号值=%#.2f，标准值=%#.2f。" ("提示"), w307, w305, w304) -> (resulting string=w308:string)  [unwired: 2 in, 1 out]
              }
            }
          }
        }
        n157 = call "Add State to Queue.vi"("State(s) In (\"\")"="init: all\nCal: Over\nidle" ("State(s) In (\"\")")) -> ("States Out"=w272:string)  [unwired: 14 in]
        n158 = global read "多参数全局变量.vi" "多参数编号"() -> (w278:string)
        n159 = Format Into String(format string="编号：%s\n参数：%s\n信息：%s" ("格式字符串"), w278, w277, w274) -> (resulting string=w275:string)  [unwired: 2 in, 1 out]
        n160 = One Button Dialog(message=w275) -> ()  [unwired: 1 in, 1 out]
        n161 = call "校准日志.vi"("table"="校准记录", "日志信息"=w275) -> ()  [unwired: 9 in, 1 out]
      }
      frame "Cal: Over" {
        n162 = global read "多参数全局变量.vi" "校准运行状态"() -> (w310:T8)
        n163 = Bundle By Name(cluster=w310, "Turb"=FALSE ("Cond")) -> (w311:T8)
        n164 = global write "多参数全局变量.vi" "校准运行状态"(w311) -> ()
      }
      frame "idle", Default {
        n165 = event shown="[8] \"校准启动\": 值改变" {
          selector: _ -> [_ _ _ _ _ _ _ _ _ _]
          dyn-events: _ -> [_ _ _ _ _ _ _ _ _ _]
          timeout: 10 -> [_ _ _ _ _ _ _ _ _ _]
          tunnel: w323 -> [w326 w330 w335 w341 w349 w357 w362 w371 w386 _]
          tunnel: [w325 w329 w336 w345 w353 w361 w364 w375 w385 w388] -> w322
          tunnel: [w324 w327 w337 w344 w352 w360 w363 w374 w383 w389] -> w321
          tunnel: w320 -> [w324 w327 w337 w344 w352 w360 w363 w374 w383 w389]
          tunnel: [_ _ _ _ _ _ _ _ w376 _] -> _
          tunnel: w316 -> [_ _ _ w339 w347 w355 _ w369 _ _]
          event Timeout {
            n166 = event-data() -> ()  [unwired: 1 in, 3 out]
            n167 = call "Add State to Queue.vi"("State(s) In (\"\")"=w326) -> ("States Out"=w325:string)  [unwired: 14 in]
          }
          event "校准模式": Value Change {
            n168 = event-data() -> ()  [unwired: 1 in, 6 out]
            n169 = call "Add State to Queue.vi"("State(s) In (\"\")"=w330, "State(s) At Back (\"\")"="init: all\nidle" ("State(s) In (\"\")")) -> ("States Out"=w329:string)  [unwired: 13 in]
          }
          event "标液1", "标液2", "标液3", "滤波设定": Mouse Down {
            n170 = event-data() -> ("CtlRef"=w334:refnum<vi>)  [unwired: 1 in, 7 out]
            n171 = property class="DigNum (严格)"(reference=w334) -> (reference out=w331:refnum<vi>, "Value"=w332:sgl)  [unwired: 1 in, 1 out]
            n172 = call "数字键盘.vi"("OldNumber"=w332) -> ("NewNumber"=w333:dbl)  [unwired: 1 in]
            n173 = property class="DigNum (严格)"(reference=w331, "Val(Sgnl)"=w333) -> ()  [unwired: 1 in, 2 out]
            n174 = call "Add State to Queue.vi"("State(s) In (\"\")"=w335) -> ("States Out"=w336:string)  [unwired: 14 in]
          }
          event "标液1": Value Change {
            n175 = event-data() -> ("NewVal"=w342:sgl)  [unwired: 1 in, 5 out]
            n176 = global read "多参数全局变量.vi" "MB session in"() -> (w343:refnum<class "MB_Master.lvclass">)
            n177 = call "纳清叶绿素a_第一点校准数据写入.vi"("数值"=w342, "MB session in"=w343) -> ("error out"=w340:errorcluster)  [unwired: 8 in, 1 out]
            n178 = Enqueue Element At Opposite End(queue=w339, element=T1."Turb" ("元素"), error in (no error)=w340) -> ()  [unwired: 1 in, 3 out]
            n179 = call "Add State to Queue.vi"("State(s) In (\"\")"=w341) -> ("States Out"=w345:string)  [unwired: 14 in]
          }
          event "标液2": Value Change {
            n180 = event-data() -> ("NewVal"=w350:sgl)  [unwired: 1 in, 5 out]
            n181 = global read "多参数全局变量.vi" "MB session in"() -> (w351:refnum<class "MB_Master.lvclass">)
            n182 = call "纳清叶绿素a_第二点校准数据写入.vi"("数值"=w350, "MB session in"=w351) -> ("error out"=w348:errorcluster)  [unwired: 8 in, 1 out]
            n183 = Enqueue Element At Opposite End(queue=w347, element=T1."Turb" ("元素"), error in (no error)=w348) -> ()  [unwired: 1 in, 3 out]
            n184 = call "Add State to Queue.vi"("State(s) In (\"\")"=w349) -> ("States Out"=w353:string)  [unwired: 14 in]
          }
          event "标液3": Value Change {
            n185 = event-data() -> ("NewVal"=w358:sgl)  [unwired: 1 in, 5 out]
            n186 = global read "多参数全局变量.vi" "MB session in"() -> (w359:refnum<class "MB_Master.lvclass">)
            n187 = call "纳清叶绿素a_第三点校准数据写入.vi"("数值"=w358, "MB session in"=w359) -> ("error out"=w356:errorcluster)  [unwired: 8 in, 1 out]
            n188 = Enqueue Element At Opposite End(queue=w355, element=T1."Turb" ("元素"), error in (no error)=w356) -> ()  [unwired: 1 in, 3 out]
            n189 = call "Add State to Queue.vi"("State(s) In (\"\")"=w357) -> ("States Out"=w361:string)  [unwired: 14 in]
          }
          event "滤波设定": Value Change {
            n190 = event-data() -> ()  [unwired: 1 in, 6 out]
            n191 = flat-sequence {
              frame #0 {
                n192 = global read "断电保存变量.vi" "滤波设置"() -> (w367:T4)
                n193 = local read "滤波设定"() -> (w365:sgl)
                n194 = Bundle By Name(cluster=w367, "Turb"=w365) -> (w366:T4)
                n195 = global write "断电保存变量.vi" "滤波设置"(w366) -> ()
              }
              frame #1 {
                n196 = call "配置文件保存.vi"() -> ()  [unwired: 12 in]
              }
            }
            n197 = call "Add State to Queue.vi"("State(s) In (\"\")"=w362) -> ("States Out"=w364:string)  [unwired: 14 in]
          }
          event "量程": Value Change {
            n198 = event-data() -> ("NewVal"=w372:u16)  [unwired: 1 in, 5 out]
            n199 = global read "多参数全局变量.vi" "MB session in"() -> (w373:refnum<class "MB_Master.lvclass">)
            n200 = call "纳清浊度_量程写入.vi"("数值"=w372, "MB session in"=w373) -> ("error out"=w370:errorcluster)  [unwired: 8 in, 1 out]
            n201 = Enqueue Element At Opposite End(queue=w369, element=T1."Turb" ("元素"), error in (no error)=w370) -> ()  [unwired: 1 in, 3 out]
            n202 = call "Add State to Queue.vi"("State(s) In (\"\")"=w371) -> ("States Out"=w375:string)  [unwired: 14 in]
          }
          event "校准启动": Value Change {
            n203 = event-data() -> ()  [unwired: 1 in, 6 out]
            n204 = global read "纳清过程全局变量.vi" "浊度测试值"() -> (w378:T3)
            n205 = Unbundle By Name(w378) -> ("量程"=w377:u16)
            n206 = global read "多参数全局变量.vi" "MB session in"() -> (w379:refnum<class "MB_Master.lvclass">)
            n207 = call "纳清浊度_校准量程写入.vi"("数值"=w377, "MB session in"=w379) -> ("error out"=w376:errorcluster)  [unwired: 8 in, 1 out]
            n208 = global read "多参数全局变量.vi" "校准运行状态"() -> (w381:T8)
            n209 = Bundle By Name(cluster=w381, "Turb"=TRUE ("Cond")) -> (w382:T8)
            n210 = global write "多参数全局变量.vi" "校准运行状态"(w382) -> ()
            n211 = call "Add State to Queue.vi"("State(s) In (\"\")"=w386, "State(s) At Back (\"\")"="init: all\nCal: Place standard solution\n Cal: Calibration process\nidle" ("State(s) In (\"\")")) -> ("States Out"=w385:string)  [unwired: 13 in]
          }
          event "校准停止": Value Change {
            n212 = event-data() -> ()  [unwired: 1 in, 6 out]
            n213 = call "Add State to Queue.vi"("State(s) In (\"\")"="init: all\nCal: Over\nidle" ("State(s) In (\"\")")) -> ("States Out"=w388:string)  [unwired: 14 in]
          }
        }
      }
    }
  }
